vi "Vision Processing.vi"(4 "error in (no error)":errorcluster, 7 "Image Size":T1=enum."320x240") -> ()   [LabVIEW 2015]
doc: "This VI runs in parallel to other tasks. It gets images from the camera, processes them for color or shape and use that information to affect robot behavior."
uses:
  <vilib>/Rock Robotics/WPI/Camera/WPI_CameraImageSize.ctl
  <vilib>/Rock Robotics/WPI/Camera/WPI_CameraWhite Balance Values.ctl
  <vilib>/Rock Robotics/WPI/Camera/WPI_CameraFrameRate.ctl
  <vilib>/Rock Robotics/WPI/Camera/WPI_CameraExposure Values.ctl
  Robot Global Data.vi
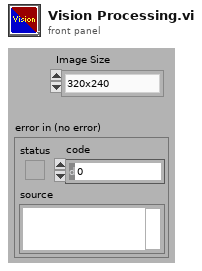
[diagram p1: front panel]
types:
  T1 = typedef "WPI_CameraImageSize.ctl" = enum16{"640x480", "320x240", "160x120", "Custom"}
  T2 = typedef "WPI_CameraFrameRate.ctl" = u32
  T3 = typedef "WPI_CameraWhite Balance Values.ctl" = enum16{"Auto", "Fixed indoor", "Fixed outdoor 1", "Fixed outdoor 2", "Fixed fluorescent 1", "Fixed fluorescent 2", "Hold current", "Custom"}
  T4 = typedef "WPI_CameraDevRef.ctl" = cluster{"Camera Address":string, "CameraStatus":errorcluster}
  T5 = typedef "WPI_CameraExposure Values.ctl" = enum16{"Auto", "Flicker-free 50 Hz", "Flicker-free 60 Hz", "Hold current", "Custom"}
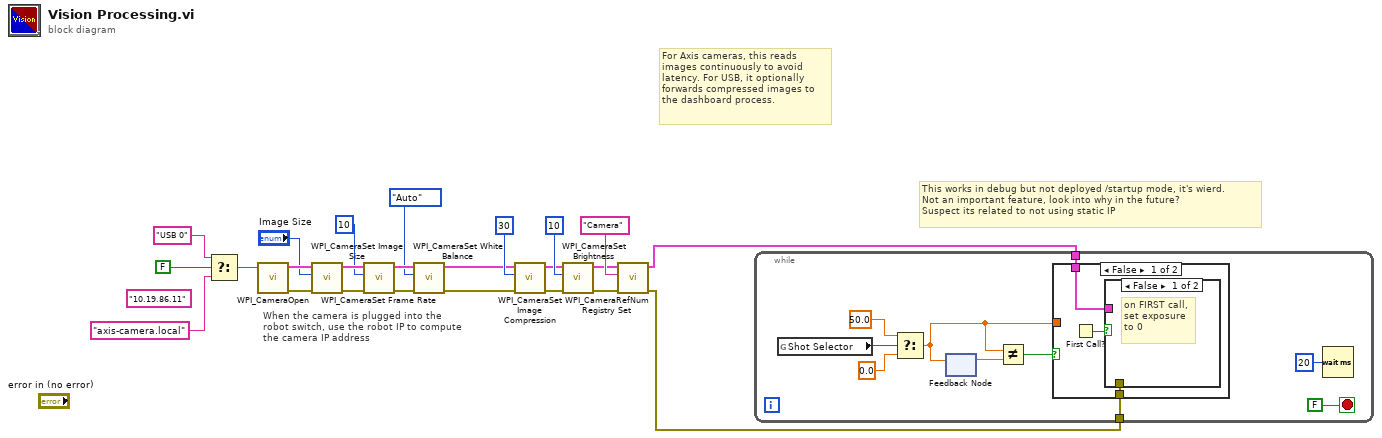
[diagram p0: block diagram]
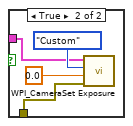
[diagram p2: hidden frame]
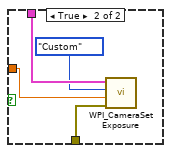
[diagram p3: hidden frame]
diagram:
  (unwired) "10.19.86.11" ("format string")
  # "This works in debug but not deployed /startup mode, it's wierd. \nNot an important feature, look into why in the future?\nSuspect its related to not using static IP"
  # "For Axis cameras, this reads\nimages continuously to avoid\nlatency. For USB, it optionally\nforwards compressed images to\nthe dashboard process."
  # "When the camera is plugged into the\nrobot switch, use the robot IP to compute\nthe camera IP address"
  n1 = Select(t="USB 0" ("format string"), s=FALSE ("dot notation? (F)"), f="axis-camera.local" ("format string")) -> (s? t:f=w6:string)
  n2 = call <vilib>:"WPI_CameraOpen.vi"("Camera Address"=w6) -> ("error out"=w17:errorcluster, "CameraDevRef"=w18:T4)  [unwired: 1 in, 8 out]
  n3 = call <vilib>:"WPI_CameraSet Image Size.vi"("error in (no error)"=w17, "Image Size"="Image Size", "CameraDevRef"=w18) -> ("error out"=w16:errorcluster, "CameraDevRef Out"=w19:T4)  [unwired: 1 in, 6 out]
  n4 = call <vilib>:"WPI_CameraSet Frame Rate.vi"("error in (no error)"=w16, "Frame Rate (fps)"=T2 10, "CameraDevRef"=w19) -> ("error out"=w15:errorcluster, "CameraDevRef Out"=w20:T4)  [unwired: 7 out]
  n5 = call <vilib>:"WPI_CameraSet White Balance.vi"("error in (no error)"=w15, "White Balance"=WPI_CameraWhite_Balance_Values."Auto", "CameraDevRef"=w20) -> ("error out"=w4:errorcluster, "CameraDevRef Out"=w5:T4)  [unwired: 1 in, 6 out]
  n6 = call <vilib>:"WPI_CameraSet Image Compression.vi"("error in (no error)"=w4, "Compression"=30, "CameraDevRef"=w5) -> ("error out"=w14:errorcluster, "CameraDevRef Out"=w21:T4)  [unwired: 7 out]
  n7 = call <vilib>:"WPI_CameraSet Brightness.vi"("error in (no error)"=w14, "Brightness"=10, "CameraDevRef"=w21) -> ("error out"=w12:errorcluster, "CameraDevRef Out"=w13:T4)  [unwired: 7 out]
  n8 = call <vilib>:"WPI_CameraRefNum Registry Set.vi"("error in (no error)"=w12, "refnum name"="Camera", "CameraDevRef"=w13) -> ("error out"=w3:errorcluster, "CameraDevRef"=w1:T4)  [unwired: 1 in, 6 out]
  n9 = while {
    tunnel: w1 -> [w26]
    tunnel: w3 -> [w25]
    stop <- FALSE stop-if-true
    n10 = global read "Robot Global Data.vi" "Shot Selector"() -> (w33:bool)
    n11 = Select(t=50.0, s=w33, f=0.0) -> (s? t:f=w28:dbl)
    n12 = feedback-in #1(w28) -> ()
    n13 = feedback #1() -> (w30:dbl)  [unwired: 1 in]
    n14 = Not Equal?(x=w28, y=w30) -> (x != y?=w29:bool)
    n15 = case shown="False" w29 {
      tunnel: w28 -> [_ w43]
      tunnel: w26 -> [w36 w45]
      tunnel: w25 -> [w35 w44]
      frame False {
        n16 = First Call?() -> (First Call?: T/F=w37:bool)
        n17 = case shown="False" w37 {
          tunnel: w36 -> [_ w40]
          tunnel: w35 -> [_ w39]
          frame False {
            # "on FIRST call,\nset exposure\nto 0"
          }
          frame True {
            n18 = call <vilib>:"WPI_CameraSet Exposure.vi"("error in (no error)"=w39, "Exposure (%)"=0.0, "Exposure"=WPI_CameraExposure_Values."Custom", "CameraDevRef"=w40) -> ()  [unwired: 8 out]
          }
        }
      }
      frame True {
        n19 = call <vilib>:"WPI_CameraSet Exposure.vi"("error in (no error)"=w44, "Exposure (%)"=w43, "Exposure"=WPI_CameraExposure_Values."Custom", "CameraDevRef"=w45) -> ()  [unwired: 8 out]
      }
    }
    n20 = Wait (ms)(milliseconds to wait=u32 20) -> ()  [unwired: 1 out]
  }
